vi "Quick Start - Run - Create.vi"() -> ()   [LabVIEW 2020]
uses:
  Nominal Client/Nominal Client.lvclass
  19192e5f-c46e-4483-8f4d-33940d6cf31d.vi
  Run/Run.lvclass
panel:
  out "rid":string
  in  "Titles":cluster{"Name":string, "Description":string}
  in  "Timing":cluster{"Start":timestamp, "End":timestamp} {"End" format="%<%x %.3X>T"; "Start" format="%<%x %.3X>T"}
  in  "Additional Configuration":T1
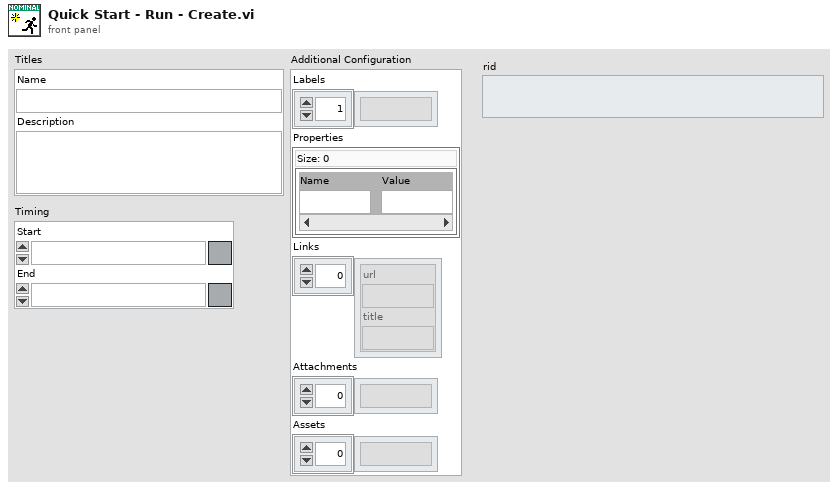
[diagram p1: front panel]
types:
  T1 = cluster{"Labels":string[], "Properties":map{string, string}, "Links":cluster{"url":string, "title":string}[], "Attachments":string[], "Assets":string[]}
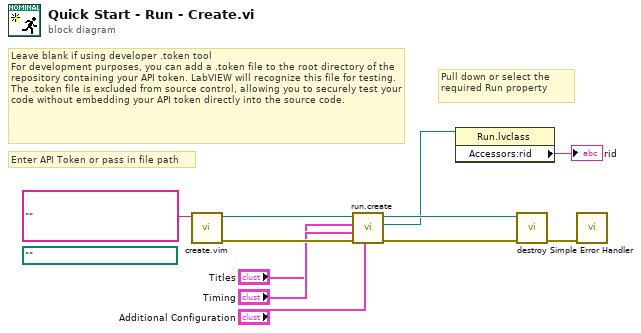
[diagram p0: block diagram]
diagram:
  (unwired) path ""
  # "Pull down or select the required Run property"
  # "Leave blank if using developer .token tool\nFor development purposes, you can add a .token file to the root directory of the repository containing your API token. LabVIEW will recognize this file for testing. The .token file is excluded from source control, allowing you to securely test your code without embedding your API token directly into the source code."
  # "Enter API Token or pass in file path"
  n1 = call "create.vim"("API Token (string or path)"="" ("API Token")) -> ("error out"=w9:errorcluster, "Nominal Client"=w10:refnum<class "Nominal Client.lvclass">)  [unwired: 9 in]
  n2 = call "run.create.vi"(6:"Additional Configuration", "error in"=w9, "Start Time (now)"="Timing", "Title"="Titles", "Nominal Client in"=w10) -> ("error out"=w8:errorcluster, "Run"=w2:refnum<class "Run.lvclass">, "Nominal Client out"=w7:refnum<class "Nominal Client.lvclass">)  [unwired: 4 in]
  n3 = property class="Run.lvclass"(reference=w2) -> ("Accessors:rid"=→"rid":string)  [unwired: 1 in, 2 out]
  n4 = call "destroy.vi"("error in"=w8, "Nominal Client"=w7) -> ("error out"=w3:errorcluster)  [unwired: 9 in]
  n5 = call <vilib>:"Simple Error Handler.vi"("error in (no error)"=w3) -> ()  [unwired: 4 in, 5 out]
